vi ".NET Type Builder Define Struct.vi"(8 "error in (no error)":errorcluster, 9 "Pack Size":i32(ring)=8 items=["Unspecified"=0, "Size1"=1, "Size2"=2, "Size4"=4, "Size8"=8, "Size16"=16, "Size32"=32, "Size64"=64, "Size128"=128], 10 "Name":string) -> (0 "error out":errorcluster, 1 ".NET Type Builder":refnum<k24>)   [LabVIEW 2018, in "TwinCAT ADS.lvclass"]
uses:
  TwinCAT ADS.lvclass
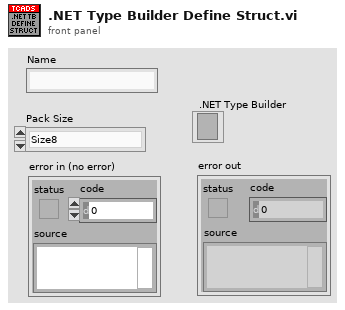
[diagram p1: front panel]
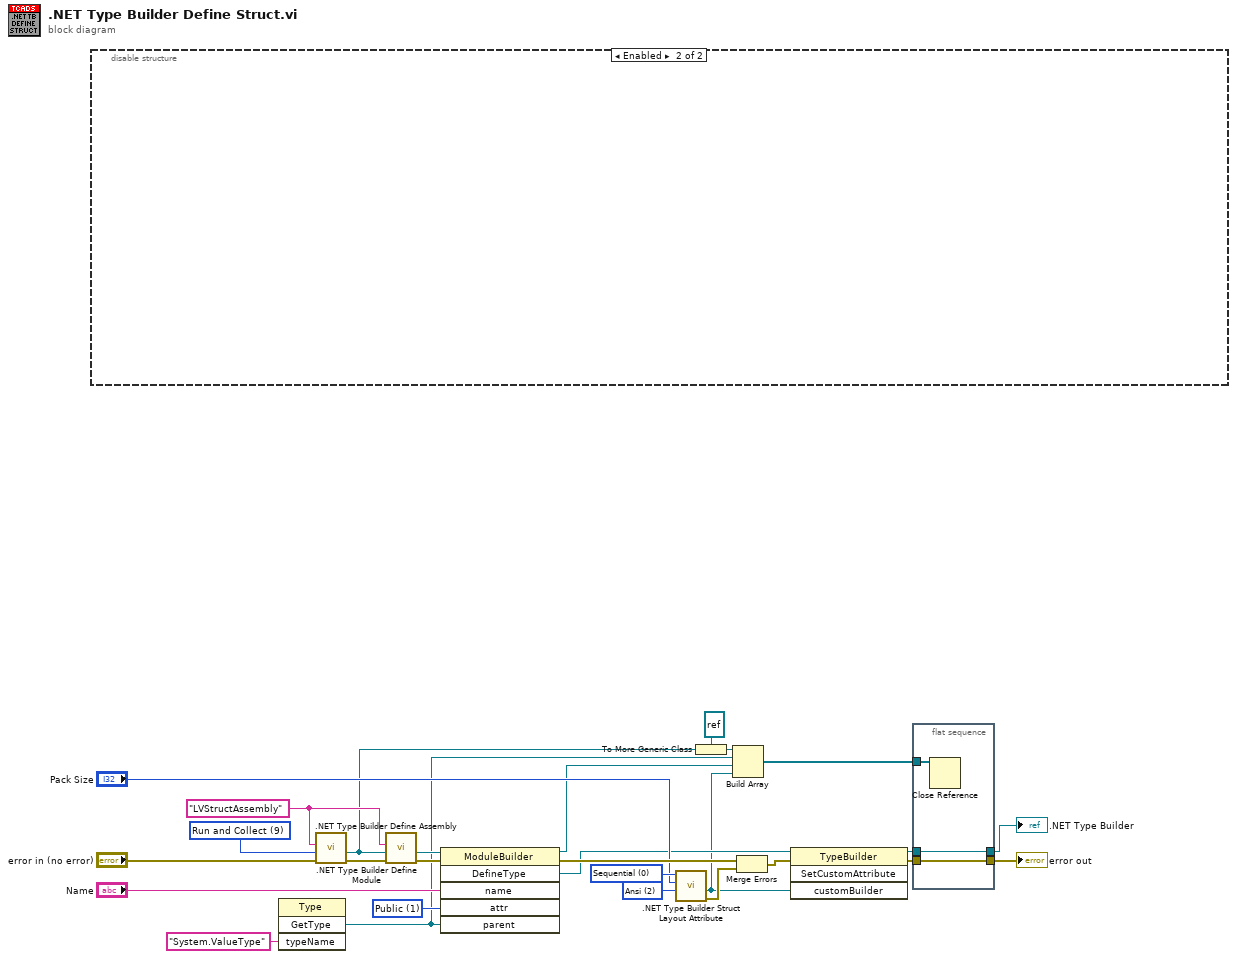
[diagram p0: block diagram]
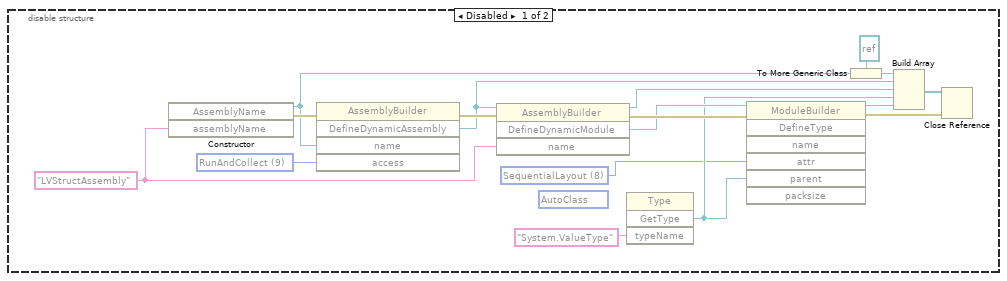
[diagram p2: hidden frame]
diagram:
  w12 = 0 items=["Sequential"=0, "Explicit"=2, "Auto"=3] ("Layout Kind")
  w13 = 2 items=["None"=1, "Ansi"=2, "Unicode"=3, "Auto"=4] ("Char Set")
  w16 = 1 items=["NotPublic, AutoLayout, AnsiClass, Class"=0, "Public"=1, "NestedPublic"=2, "NestedPrivate"=3, "NestedFamily"=4, "NestedAssembly"=5, "NestedFamANDAssem"=6, "NestedFamORAssem, VisibilityMask"=7, "SequentialLayout"=8, "ExplicitLayout"=16, "LayoutMask"=24, "Interface, ClassSemanticsMask"=32, "Abstract"=128, "Sealed"=256, "SpecialName"=1024, "RTSpecialName"=2048, "Import"=4096, "Serializable"=8192, "WindowsRuntime"=16384, "UnicodeClass"=65536, "AutoClass"=131072, "StringFormatMask, CustomFormatClass"=196608, "HasSecurity"=262144, "ReservedMask"=264192, "BeforeFieldInit"=1048576, "CustomFormatMask"=12582912] ("attr")
  w20 = "LVStructAssembly" ("assemblyName")
  w21 = 9 items=["Run"=1, "Save"=2, "Run and Save"=3, "Reflection Only"=6, "Run and Collect"=9] ("Access (Run and Collect)")
  n1 = disable-structure shown="Enabled" {
    frame Disabled {
      (unwired) 131072 items=["NotPublic, AutoLayout, AnsiClass, Class"=0, "Public"=1, "NestedPublic"=2, "NestedPrivate"=3, "NestedFamily"=4, "NestedAssembly"=5, "NestedFamANDAssem"=6, "NestedFamORAssem, VisibilityMask"=7, "SequentialLayout"=8, "ExplicitLayout"=16, "LayoutMask"=24, "Interface, ClassSemanticsMask"=32, "Abstract"=128, "Sealed"=256, "SpecialName"=1024, "RTSpecialName"=2048, "Import"=4096, "Serializable"=8192, "WindowsRuntime"=16384, "UnicodeClass"=65536, "AutoClass"=131072, "StringFormatMask, CustomFormatClass"=196608, "HasSecurity"=262144, "ReservedMask"=264192, "BeforeFieldInit"=1048576, "CustomFormatMask"=12582912] ("attr")
      w29 = 8 items=["NotPublic, AutoLayout, AnsiClass, Class"=0, "Public"=1, "NestedPublic"=2, "NestedPrivate"=3, "NestedFamily"=4, "NestedAssembly"=5, "NestedFamANDAssem"=6, "NestedFamORAssem, VisibilityMask"=7, "SequentialLayout"=8, "ExplicitLayout"=16, "LayoutMask"=24, "Interface, ClassSemanticsMask"=32, "Abstract"=128, "Sealed"=256, "SpecialName"=1024, "RTSpecialName"=2048, "Import"=4096, "Serializable"=8192, "WindowsRuntime"=16384, "UnicodeClass"=65536, "AutoClass"=131072, "StringFormatMask, CustomFormatClass"=196608, "HasSecurity"=262144, "ReservedMask"=264192, "BeforeFieldInit"=1048576, "CustomFormatMask"=12582912] ("attr")
      w48 = 9 items=["Run"=1, "Save"=2, "RunAndSave"=3, "ReflectionOnly"=6, "RunAndCollect"=9] ("access")
      w45 = "LVStructAssembly" ("assemblyName")
      n2 = constructor class="AssemblyName"("assemblyName"=w45) -> (reference out=w38:refnum<k24>, error in=w28:errorcluster, error out=w47:errorcluster)  [unwired: 2 in, 2 out]
      n3 = invoke class="AssemblyBuilder" method="DefineDynamicAssembly"(error in=w47, "name"=w38, "access"=w48) -> (error out=w46:errorcluster, "DefineDynamicAssembly"=w37:refnum<k24>)  [unwired: 2 in, 3 out]
      n4 = invoke class="AssemblyBuilder" method="DefineDynamicModule"(reference=w37, error in=w46, "name"=w45) -> (reference out=w35:refnum<k24>, error out=w44:errorcluster, "DefineDynamicModule"=w36:refnum<k24>)  [unwired: 1 in, 1 out]
      n5 = invoke class="Type" method="GetType"("typeName"="System.ValueType") -> ("GetType"=w34:refnum<k24>)  [unwired: 3 in, 3 out]
      n6 = invoke class="ModuleBuilder" method="DefineType"(reference=w36, error in=w44, "attr"=w29, "parent"=w34) -> (reference out=w33:refnum<k24>, error out=w32:errorcluster, "DefineType"=w30:refnum<k24>, "name"=w41:string, "packsize"=w42:i32)  [unwired: 1 in, 4 out]
      n7 = To More Generic Class(target class=refnum<k24> refnum ("DefineType"), reference=w38) -> (generic class reference=w39:refnum<k24>)
      n8 = Build Array(w39, w37, w35, w34, w33) -> (w31:refnum<k24>[])
      n9 = Close Reference(reference=w31, error in (no error)=w32) -> ()  [unwired: 1 out]
    }
    frame Enabled {
    }
  }
  n10 = invoke class="Type" method="GetType"("typeName"="System.ValueType") -> ("GetType"=w8:refnum<k24>)  [unwired: 3 in, 3 out]
  n11 = call ".NET Type Builder Define Assembly.vi"("error in (no error)"="error in (no error)", "Access (Run and Collect)"=w21, "Name"=w20) -> ("error out"=w22:errorcluster, ".NET Assembly Builder"=w9:refnum<k24>)  [unwired: 7 in]
  n12 = call ".NET Type Builder Define Module.vi"("error in (no error)"=w22, ".NET Assembly Builder"=w9, "Name"=w20) -> ("error out"=w19:errorcluster, ".NET Module Builder"=w18:refnum<k24>)  [unwired: 7 in]
  n13 = invoke class="ModuleBuilder" method="DefineType"(reference=w18, error in=w19, "name"="Name", "attr"=w16, "parent"=w8) -> (reference out=w7:refnum<k24>, error out=w27:errorcluster, "DefineType"=w6:refnum<k24>)  [unwired: 1 in, 3 out]
  n14 = call ".NET Type Builder Struct Layout Attribute.vi"("Char Set"=w13, "Pack Size"="Pack Size", "Layout Kind"=w12) -> ("error out"=w26:errorcluster, ".NET Custom Attribute Builder"=w5:refnum<k24>)  [unwired: 7 in]
  n15 = To More Generic Class(target class=refnum<k24> refnum ("DefineType"), reference=w9) -> (generic class reference=w24:refnum<k24>)
  n16 = Build Array(w24, w8, w7, w5) -> (w23:refnum<k24>[])
  n17 = Merge Errors(w27, w26) -> (w10:errorcluster)
  n18 = invoke class="TypeBuilder" method="SetCustomAttribute"(reference=w6, error in=w10, "customBuilder"=w5) -> (reference out=w4:refnum<k24>, error out=w3:errorcluster)  [unwired: 1 in, 2 out]
  n19 = flat-sequence {
    tunnel: w23 -> [w51]
    tunnel: w4 -> [w49]
    tunnel: w3 -> [w50]
    tunnel: [w50] -> w2
    tunnel: [w49] -> w1
    frame #0 {
      n20 = Close Reference(reference=w51) -> ()  [unwired: 1 in, 1 out]
    }
  }
  "error out" <- w2
  ".NET Type Builder" <- w1
